vi "Histogram2D1005.vi"   [LabVIEW 2013]
uses:
  <vilib>/Heliosphere Research LLC/Advanced Plotting Toolkit/api_plotting/Histogram2DRange.ctl
  <vilib>/Heliosphere Research LLC/Advanced Plotting Toolkit/api_plotting/Histogram2D_Automatic.vi
  <vilib>/Heliosphere Research LLC/Advanced Plotting Toolkit/Advanced Plotting Toolkit.lvlib
types:
  T1 = typedef "Advanced Plotting Toolkit.lvlib/Histogram2DRange.ctl" = cluster{"X Min":dbl, "X Max":dbl, "Y Min":dbl, "Y Max":dbl}
  T2 = typedef "Advanced Plotting Toolkit.lvlib/PlotID.ctl" = i32
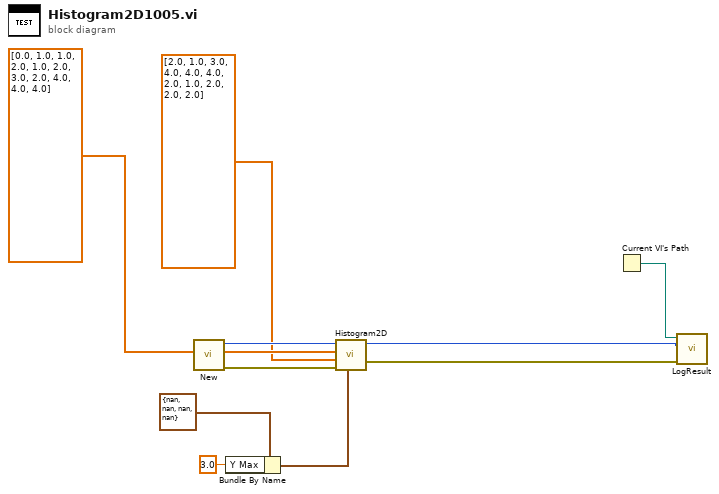
[diagram p0: block diagram]
diagram:
  n1 = call <vilib>:"New.vi"() -> ("error out"=w8:errorcluster, "Plot ID"=w9:T2)  [unwired: 10 in]
  n2 = Bundle By Name(cluster=T1 {"X Min"=nan, "X Max"=nan, "Y Min"=nan, "Y Max"=nan} ("Data Range"), "Y Max"=3.0 ("X Min")) -> (w2:T1)
  n3 = call-poly <vilib>:"Histogram2D.vi"("Data Range"=w2, "error in (no error)"=w8, "Y Data"=dbl[] [2.0, 1.0, 3.0, 4.0, 4.0, 4.0, 2.0, 1.0, 2.0, 2.0, 2.0] ("X Data"), "X Data"=dbl[] [0.0, 1.0, 1.0, 2.0, 1.0, 2.0, 3.0, 2.0, 4.0, 4.0, 4.0], "Plot ID"=w9) -> ("error out"=w6:errorcluster, "Plot ID Out"=w7:T2)  [unwired: 5 in]
  n4 = Current VI's Path() -> (path=w10:path)
  n5 = call "LogResult.vi"("Test Result"=w6, "Test Artifact"=w7, "VI Path"=w10) -> ()  [unwired: 9 in]
